vi "peaks_old.vi"(8 "error in (no error)":errorcluster, 9 "List Parameter Fit in":dbl[][](array[numeric]), 10 "List ROI in":dbl[][](array[numeric]), 11 "Spectrum In":cluster{"Locations":dbl[], "Amplitudes":dbl[]}[](array[cluster])=[{"Locations"=array[8192 elements], "Amplitudes"=array[8192 elements]}, {"Locations"=[0.7467606671708176, 1.9235641208245904, 2.29844815204634, 2.952058877083534, 3.30159027268929, 3.693510427204611, 4.0114062030881295, 5.465964569482503, 5.90533601872882, 6.405158056693529, 7.048430896937822, 7.965886489214608, 8.618241797175692, 9.551852093117594, 10.52313535167255, 11.040953037461485, 11.06991514504198, 11.223209663036432, 12.573413841890297, 13.028543500140618, 13.063940211907648, 13.079189646232502, 13.092703597511122, 13.151136366155567, 13.270484104491407, 13.336875706360313, 14.056987568841034, 14.657535881569391, 15.704563469510273, 16.589800479761752, 17.294355204547227, 18.547875406033366, 19.386017685106246, 23.796403305697343, 24.246601838900926, 24.938407230371723], "Amplitudes"=[8249.877716133802, 11327.172305519029, 56622.259938185096, 7573.210585087449, 5296.252862567521, 568942.2217447343, 85362.57126615923, 5991.635098339018, 7019.466820603001, 22054.8389595985, 7981.806397770608, 3443.0618845857953, 7232.474442522111, 1041.175508376075, 20253.913652049327, 2798.643385245958, 2822.1764574507447, 2760.065665975324, 27847.958569595598, 7072.034132274657, 7057.281156133169, 7080.033735934979, 7084.174530276932, 7080.4596184742295, 7256.269557996548, 7151.769553474873, 10957.376602343933, 8796.257531749367, 4885.946335626738, 151185.40382805822, 73397.38735258923, 16617.278737895518, 11305.024780412065, 1494.0162050533122, 1876.7337579234295, 12601.308465489856]}]) -> (0 "Error Out":errorcluster, 1 "List ROI out":dbl[][](array[numeric]), 2 "Table":string[][](table), 3 "Peaks Out":cluster{"Locations":dbl[], "Amplitudes":dbl[]}, 4 "List Parameter Fit Out":dbl[][](array[numeric]), 6 "Spectrum Fitted":cluster{"Array":dbl[], "Array":dbl[]})   [LabVIEW 2020]
uses:
  <vilib>/Utility/miscctls.llb/LVCursorListTypeDef.ctl
  b6f9e8ca-7105-a144-8367-28ac801578dd.vi
  85740291-8aab-ac43-b547-174ae308998b.vi
  01ce4f70-08cd-4644-9d74-9876cc86ca53.vi
  <vilib>/Utility/cursorutil.llb/Set Cursor (Icon Pict).vi
  control/global name path.vi
  <vilib>/Utility/Data Type/Get Array Information.vi
  <vilib>/Utility/Data Type/Get Type Information.vi
  <vilib>/Utility/file.llb/Write Delimited Spreadsheet (DBL).vi
  <vilib>/Utility/file.llb/Write Delimited Spreadsheet (string).vi
  <vilib>/Utility/file.llb/Read Delimited Spreadsheet (string).vi
  <vilib>/Utility/file.llb/Read Delimited Spreadsheet (DBL).vi
panel:
  in  "Fit":bool
  in  "mapping":u16(ring) items=["Y - Linear", "Y - Log"]
  out "CrsrList":T1(array[cluster])
  in  "Open":bool
  in  "Save":bool
  in  "eval":bool
  in  "custom":bool
  out "cluster roi":T2
  out "element":cluster{"Locations":dbl[], "Amplitudes":dbl[]}
  out "Cursor Name":string
  in  "Reset":bool
  out "Array":dbl[][](array[numeric])
  out "removing":bool
  in  "Normal":bool
  in  "Remove":bool
  in  "Cursor Icon":u16(ring)
  in  "Stop Button":bool
  out "Spectrum":cluster{"Locations":dbl[], "Amplitudes":dbl[]}[](graph)=[{"Locations"=array[8192 elements], "Amplitudes"=array[8192 elements]}, {"Locations"=[0.6846487923218129, 0.8031614293624534, 1.7242543828557408, 1.938747247460668, 2.306953300257028, 2.6210970168759666, 2.9711981229526625, 3.3277824164248653, 3.7170873790620336, 4.04405224728037, 6.436481431667202, 7.096967343713246, 7.460990586502177, 7.523333804369678, 7.617042760860395, 8.127017296174136, 8.194901838112248, 8.297705547082785, 8.30569855209705, 8.683571266368165, 9.291525652441827, 9.336316527839342, 9.702473642891427, 10.164949159251092, 10.940151266361038, 10.984300604976537, 11.073242471735028, 11.160271165263742, 11.268603021790387, 11.368683422279902, 11.476870860603926, 11.732338216351955, 11.74047488132859, 11.913527841198139, 12.313442472513525, 12.422414883693174, 12.679357859240612, 13.137181465596367, 13.560377222755834, 13.985871403462042, 14.181757913002619, 14.811990689785183, 15.123878999537014, 15.225144239474576, 15.847402751701654, 15.936506376474796, 15.997115442383588, 16.751668923733696, 17.456338945421972, 18.685517095107702, 19.565242039112338, 23.10994450808025, 23.25953036719509, 23.37377015691927, 23.439242722748002, 23.98629158276466, 24.428149293414577, 24.684829964850557, 24.772035910147434, 25.173301655535283], "Amplitudes"=[5749.475271060954, 5002.0142432044795, 4437.978004734703, 11660.526656612647, 65746.84001208292, 2894.387213953257, 9849.360532927198, 7160.035072829482, 645601.7858592308, 95492.33538323875, 14805.060779816191, 1620.7095092057602, 1146.3915335122922, 1168.4930336372568, 1322.5033864359928, 4245.563045439152, 4184.35157964611, 4422.765014063421, 4401.872906279167, 13740.871473164421, 12716.350040257696, 12964.336303896753, 16789.033949154484, 20702.823823277406, 27073.790223214626, 26827.13611017004, 26877.36292640188, 26681.744011808405, 26623.286988764616, 26394.35650952068, 26015.737537837078, 23980.0092551179, 23996.924012643343, 23101.773776484937, 20651.803398511016, 20229.386024779047, 41284.21044656313, 13637.881570622103, 8980.093476318705, 5646.466867551864, 7355.058688359613, 4885.822952660352, 292.0377308174795, 694.6108290767994, 6797.9436035222725, 6852.18604910736, 6738.9197496309225, 156943.61193784876, 77075.8593535495, 10701.96206664513, 3415.986171238152, 30.039025289396076, 37.780232933378514, 78.71549190995782, 52.215114100379424, 895.4437472888932, 1309.544166875224, 1288.517058471017, 1383.105839373177, 18123.868845544213]}]
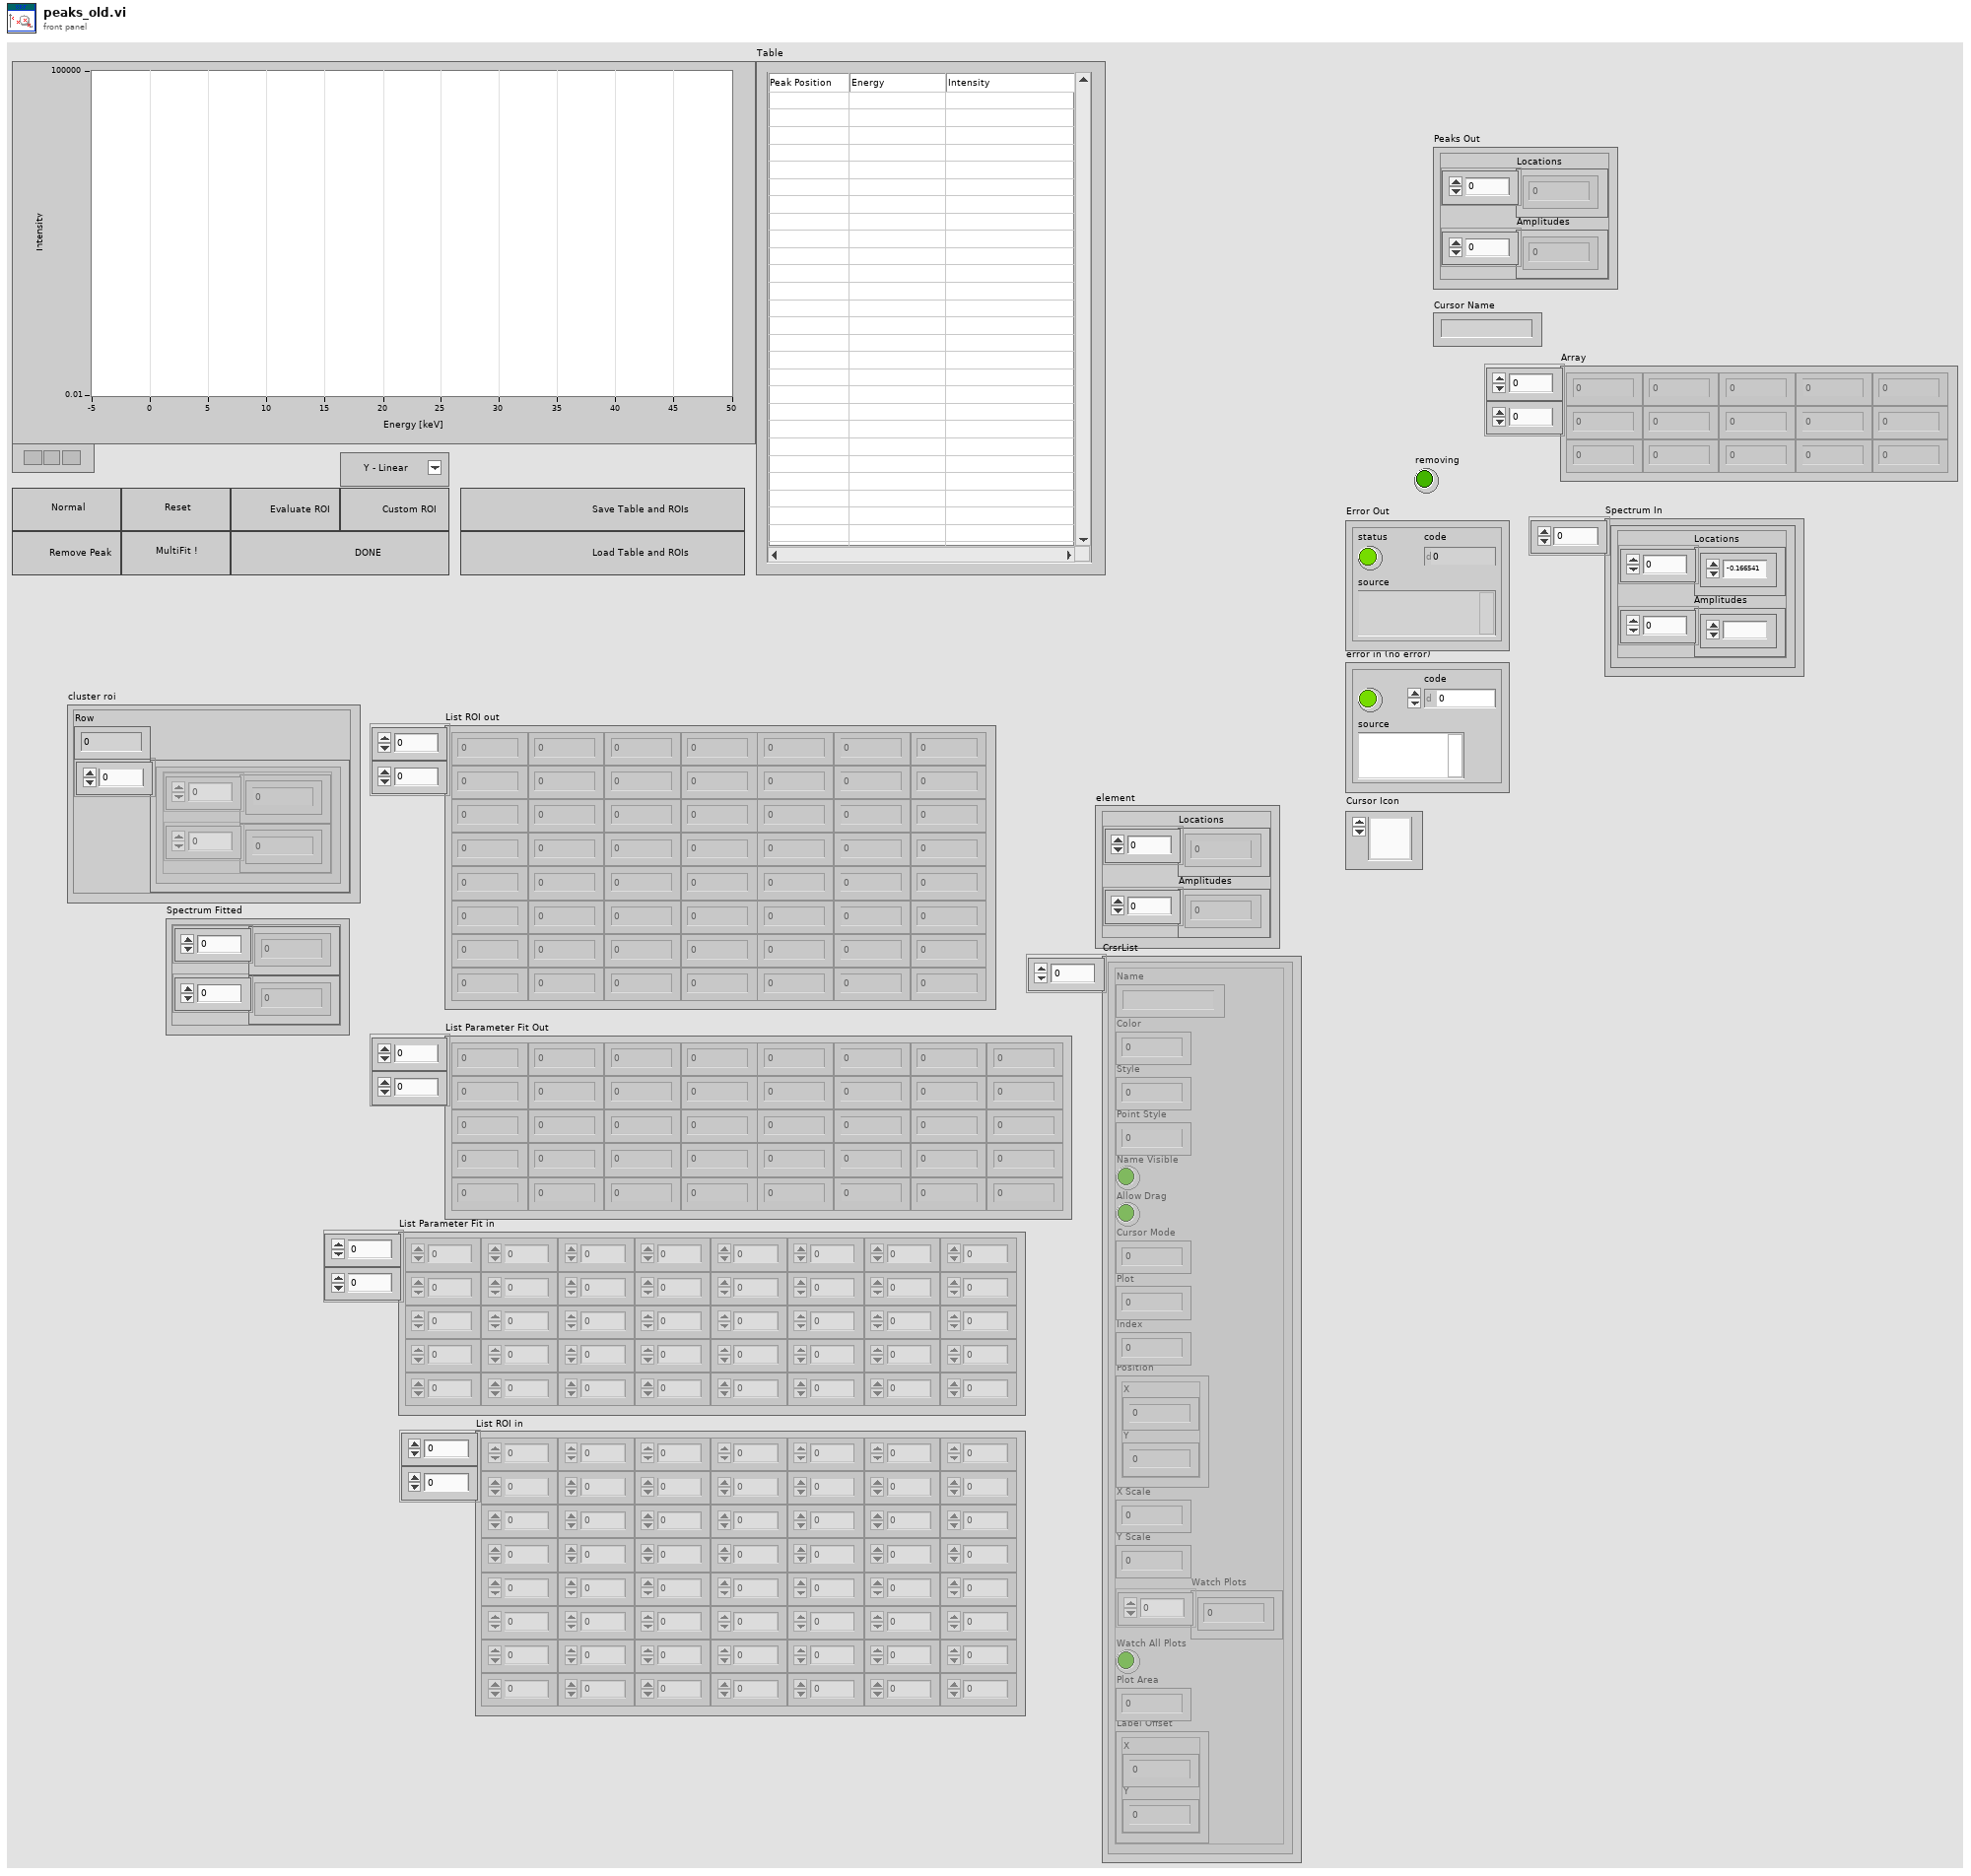
[diagram p1: front panel]
types:
  T1 = cluster{"Name":string, "Color":u32, "Style":i32, "Point Style":i32, "Name Visible":bool, "Allow Drag":bool, "Cursor Mode":u32, "Plot":i32, "Index":i32, "Position":cluster{"X":dbl, "Y":dbl}, "X Scale":u32, "Y Scale":u32, "Watch Plots":i32[], "Watch All Plots":bool, "Plot Area":i32, "Label Offset":cluster{"X":dbl, "Y":dbl}}[]
  T2 = cluster{"Row":i32, "Array":cluster{"Array":dbl[], "Array":dbl[]}[]}
  T3 = typedef "LVCursorListTypeDef.ctl" = cluster{"Name":string, "Color":u32, "Style":u8, "Point Style":u8, "Name Visible":bool, "Allow Drag":bool, "Cursor Mode":u32, "Plot":i32, "Index":i32, "Position":cluster{"X":dbl, "Y":dbl}, "X Scale":u32, "Y Scale":u32, "Watch Plots":i32[], "Watch All Plots":bool, "Plot Area":i32, "Label Offset":cluster{"X":dbl, "Y":dbl}}[]
  T4 = cluster{"Name":string, "Color":u32, "Style":i32, "Point Style":i32, "Name Visible":bool, "Allow Drag":bool, "Cursor Mode":u32, "Plot":i32, "Index":i32, "Position":cluster{"X":dbl, "Y":dbl}, "X Scale":u32, "Y Scale":u32, "Watch Plots":i32[], "Watch All Plots":bool, "Plot Area":i32, "Label Offset":cluster{"X":dbl, "Y":dbl}}
  T5 = typedef "LVPoint32TypeDef.ctl" = cluster{"Horizontal":i32, "Vertical":i32}
  T6 = typedef "LVRowAndColumnTypeDef.ctl" = cluster{"Row":i32, "Column":i32}
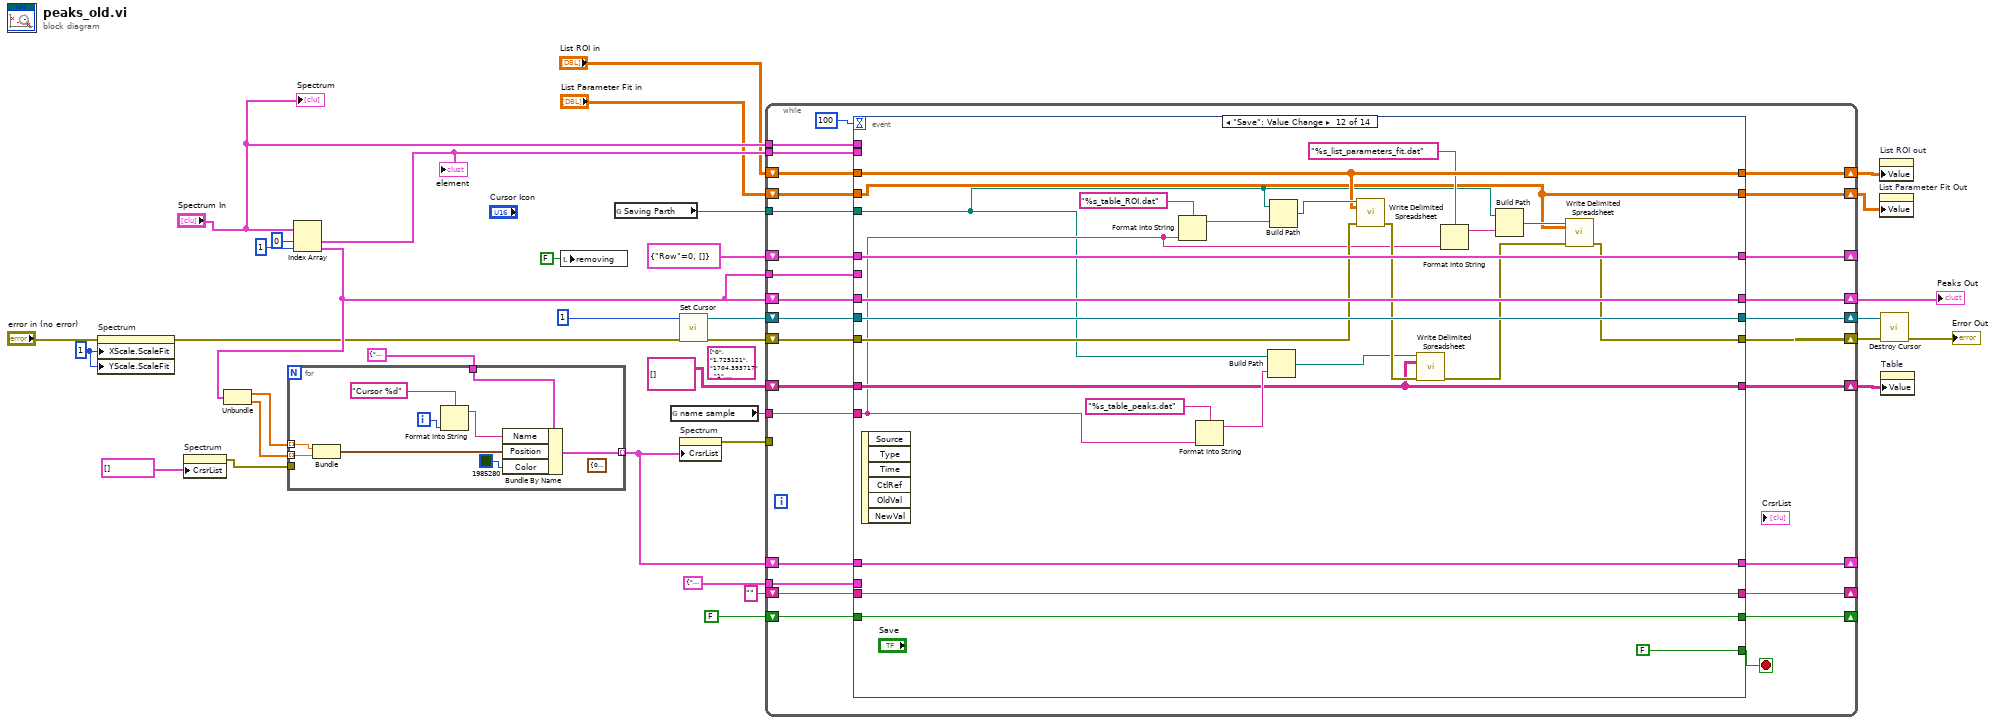
[diagram p0: block diagram]
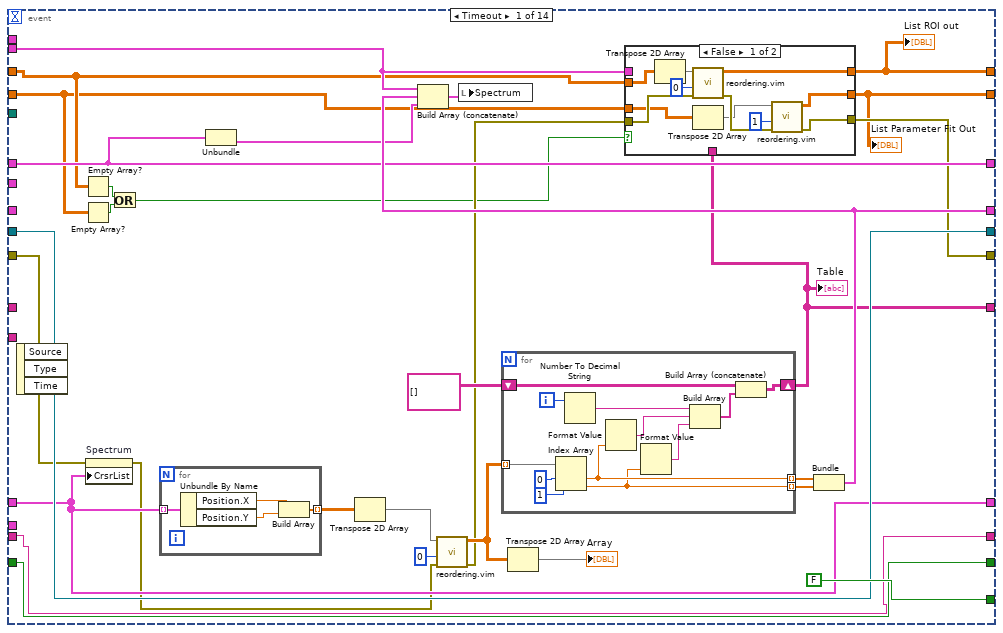
[diagram p2: hidden frame]
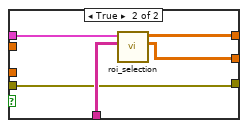
[diagram p3: hidden frame]
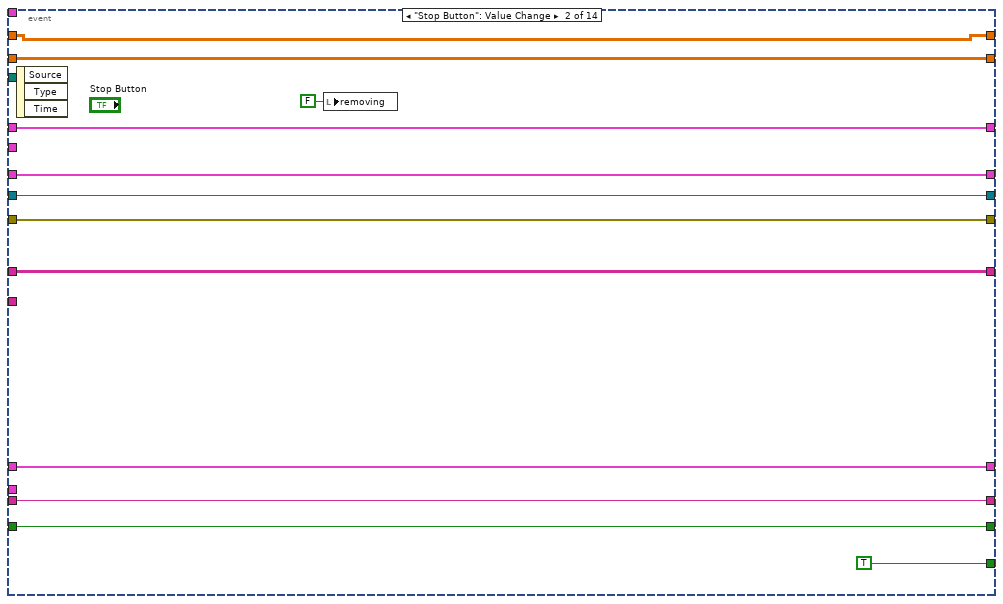
[diagram p4: hidden frame]
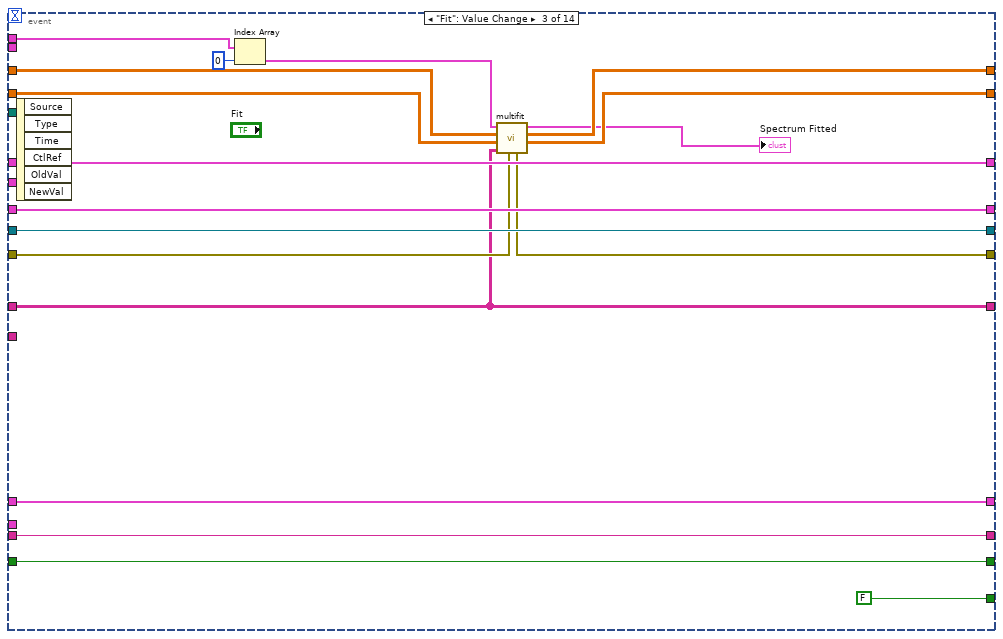
[diagram p5: hidden frame]
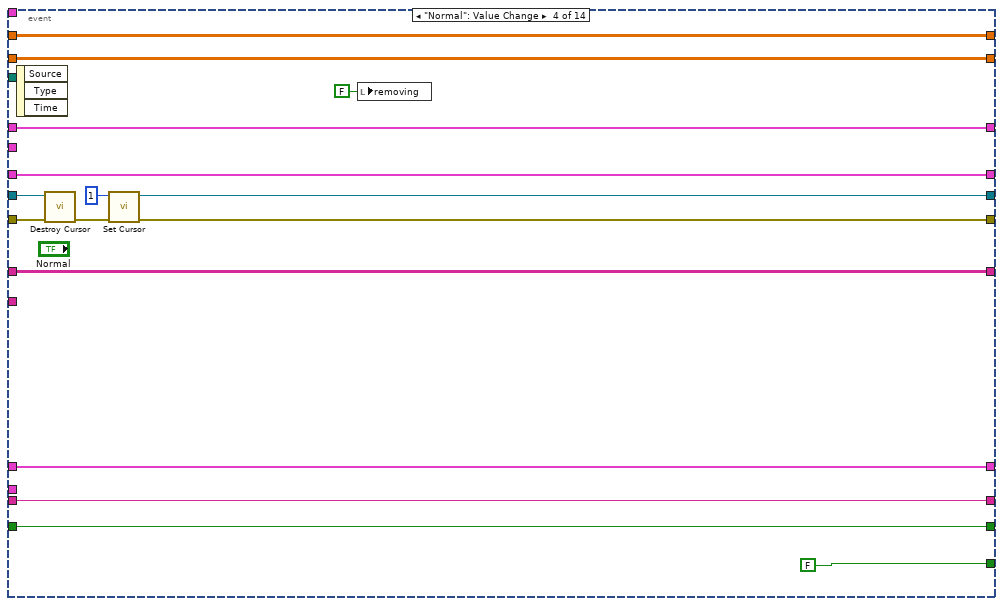
[diagram p6: hidden frame]
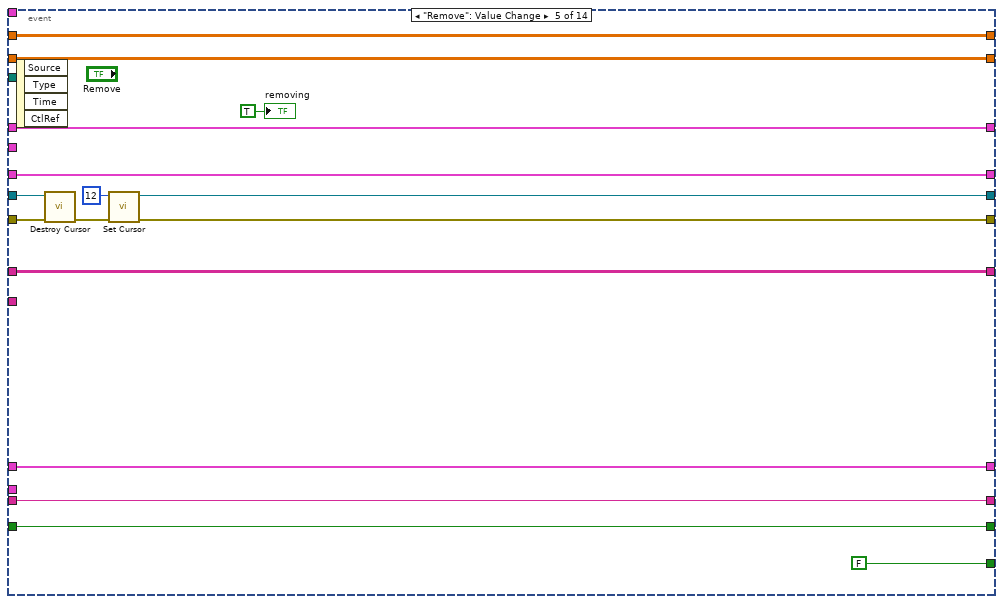
[diagram p7: hidden frame]
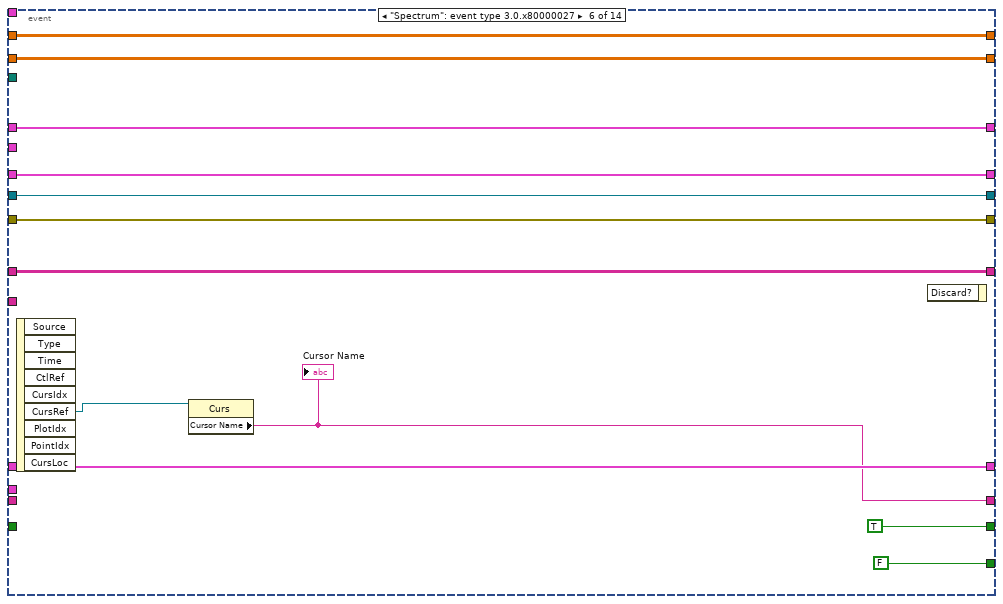
[diagram p8: hidden frame]
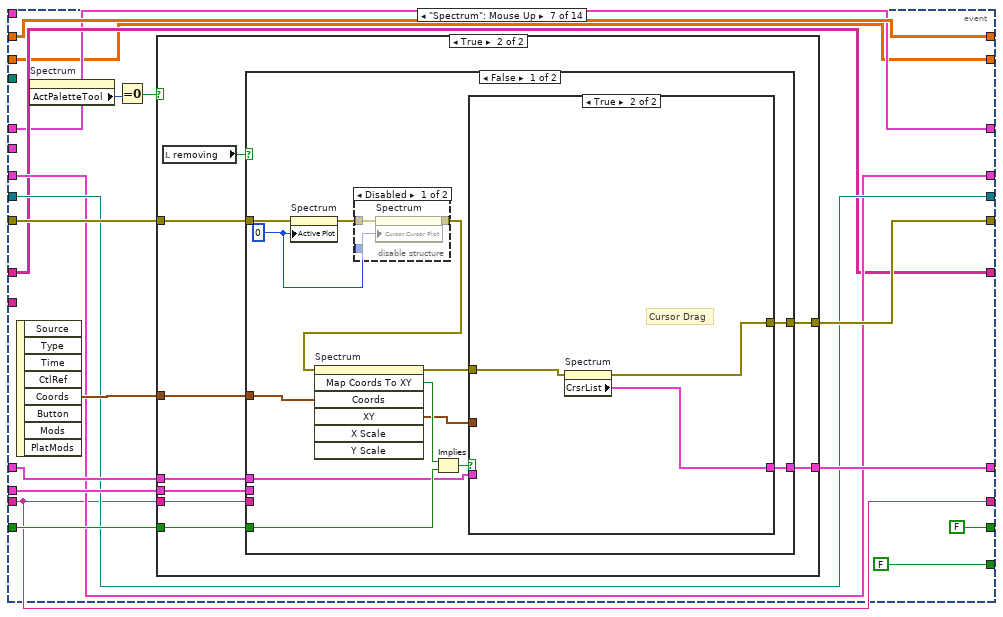
[diagram p9: hidden frame]
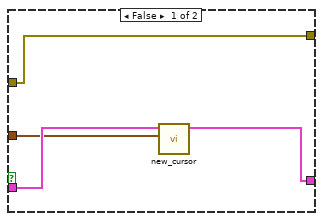
[diagram p12: hidden frame]
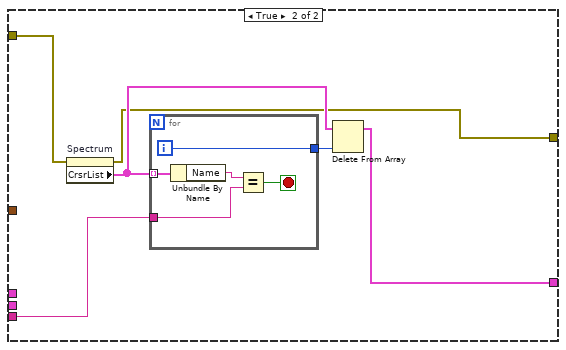
[diagram p13: hidden frame]
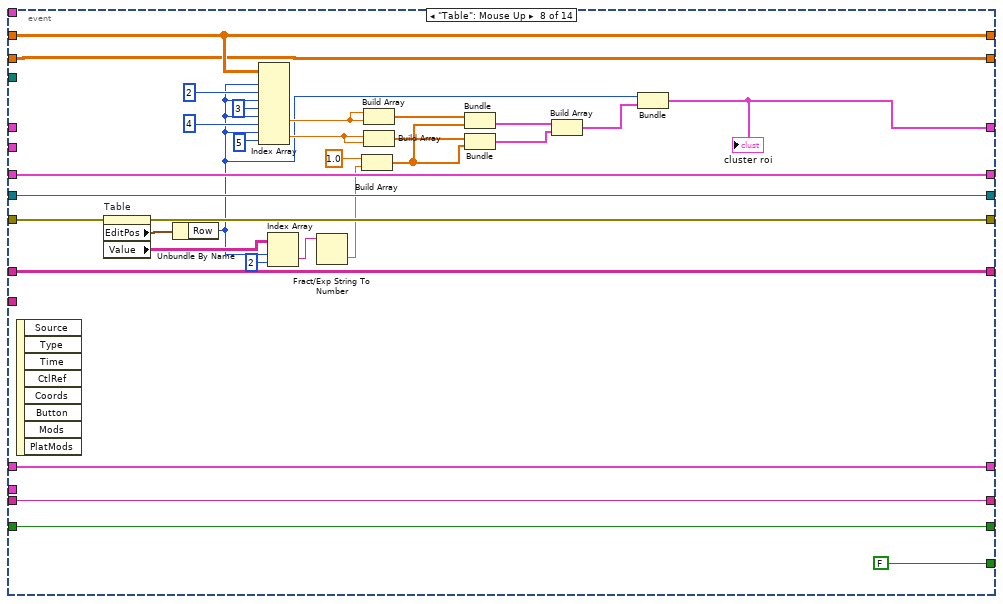
[diagram p14: hidden frame]
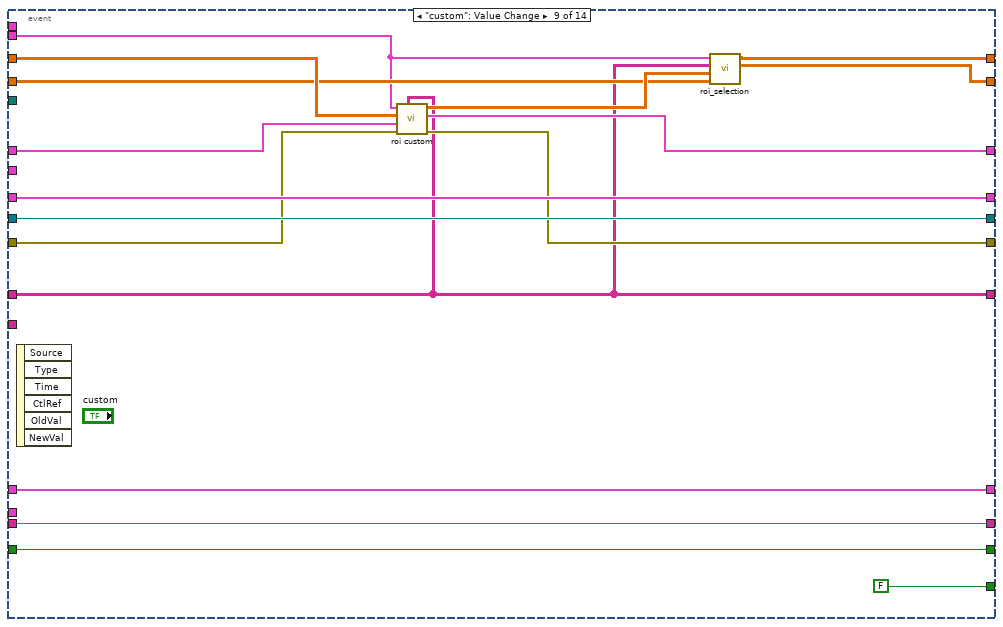
[diagram p15: hidden frame]
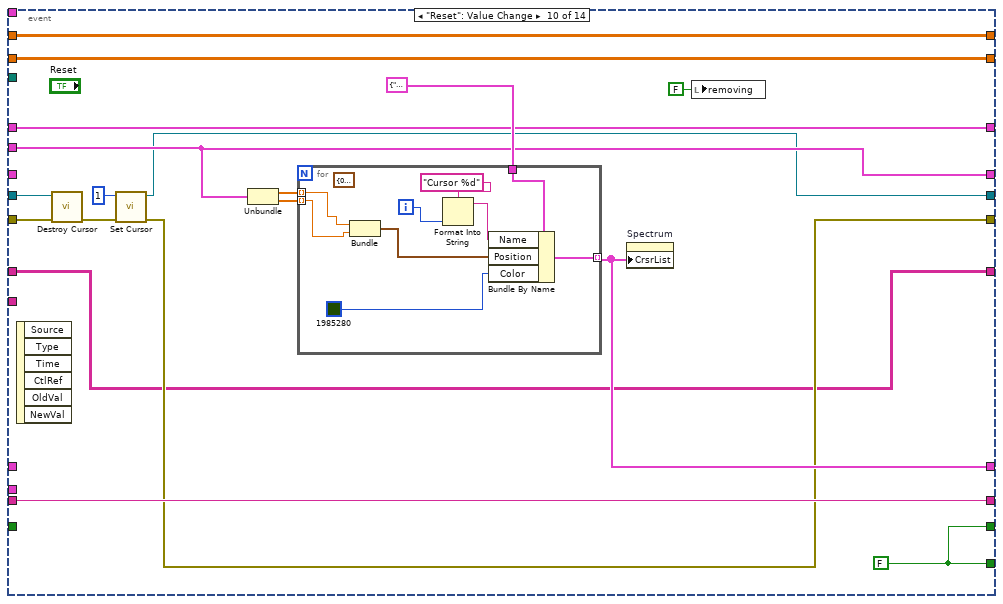
[diagram p16: hidden frame]
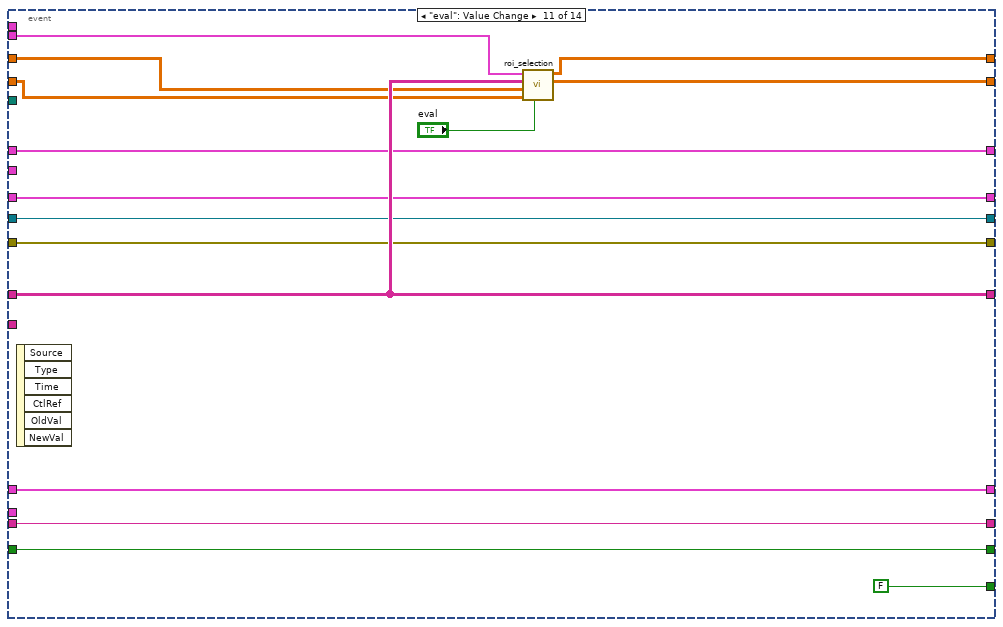
[diagram p17: hidden frame]
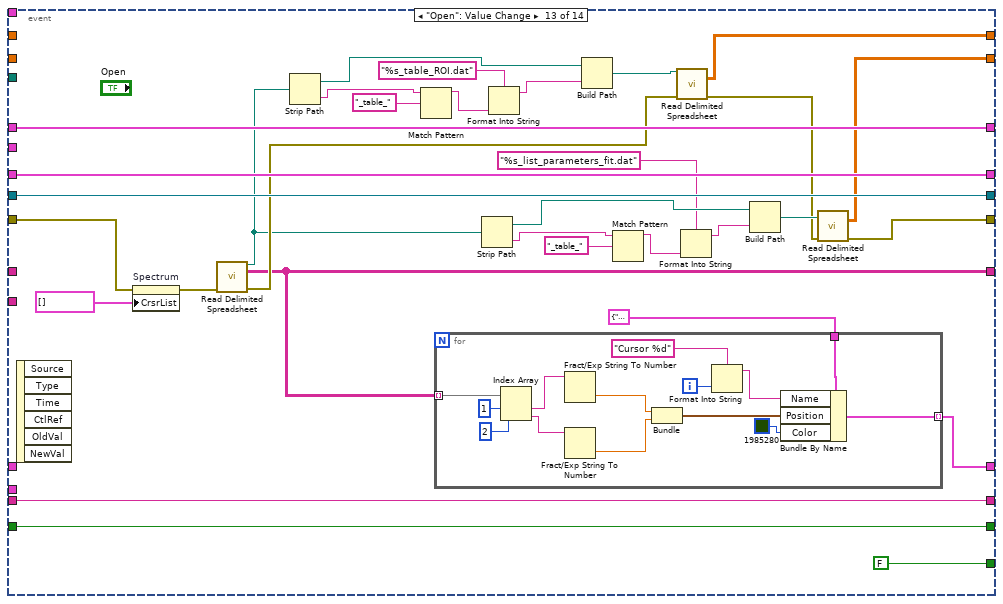
[diagram p18: hidden frame]
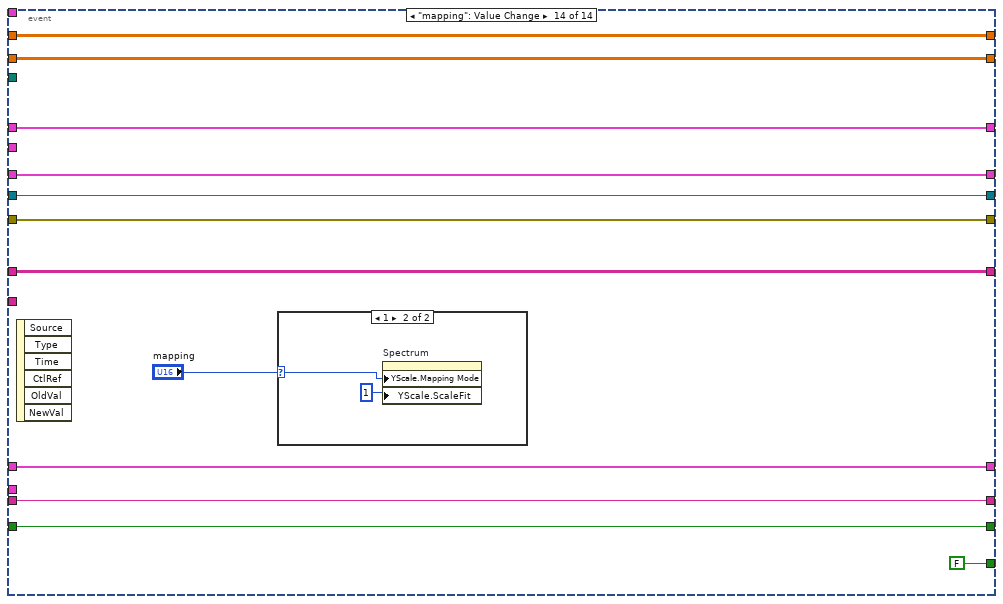
[diagram p19: hidden frame]
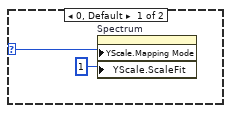
[diagram p20: hidden frame]
diagram:
  w11 = u8 1 ("X Scale.Scale Fit")
  (unwired) string[][] [["0", "1.725121", "1704.393717"], ["1", "1.970845", "984.228481"], ["2", "2.303441", "1944.031171"], ["3", "2.614035", "2011.669918"], ["4", "2.952544", "4620.007915"], ["5", "3.307548", "9783.329806"], ["6", "3.691265", "30769.779466"], ["7", "4.014453", "4616.583275"], ["8", "4.510204", "698.422233"], ["9", "4.927114", "412.615986"], ["10", "5.950437", "698.422233"], ["11", "6.402564", "4117.128631"], ["12", "8.072886", "984.228481"], ["13", "8.615424", "2806.402012"], ["14", "10.509461", "8738.084886"], ["15", "12.556457", "12119.486590"], ["16", "14.027261", "5340.202284"], ["17", "14.636488", "4362.343076"]] ("Table")
  n1 = property on="Spectrum" class="XYGraph (strict)"(error in="error in (no error)", "XScale.ScaleFit"=w11, "YScale.ScaleFit"=w11) -> (error out=w9:errorcluster)  [unwired: 1 in, 1 out]
  n2 = property on="Spectrum" class="XYGraph (strict)"("CrsrList"=T3 [] ("Cursor List")) -> (error out=w21:errorcluster)  [unwired: 2 in, 1 out]
  n3 = Index Array(array="Spectrum In", index #1=0 ("index"), index #2=1 ("index")) -> (element #1=w15:cluster{"Locations":dbl[], "Amplitudes":dbl[]}, element #2=w17:cluster{"Locations":dbl[], "Amplitudes":dbl[]})
  "element" <- w15
  n4 = Unbundle(w17) -> ("Locations"=w25:dbl[], "Amplitudes"=w24:dbl[])
  n5 = for {
    tunnel: w25 -> [w42] mode=indexing
    tunnel: w24 -> [w41] mode=indexing
    tunnel: T4 {"Name"="", "Color"=16776704, "Style"=4, "Point Style"=13, "Name Visible"=FALSE, "Allow Drag"=TRUE, "Cursor Mode"=0, "Plot"=0, "Index"=0, "Position"={"X"=0.0, "Y"=0.0}, "X Scale"=0, "Y Scale"=0, "Watch Plots"=[], "Watch All Plots"=FALSE, "Plot Area"=0, "Label Offset"={"X"=0.0, "Y"=0.0}} -> [w40]
    tunnel: w21 -> [_]
    tunnel: [w36] -> w18 mode=indexing
    i -> [w43]
    (unwired) cluster{"X":dbl, "Y":dbl} {"X"=0.0, "Y"=0.0} ("XY")
    n6 = Bundle("Numeric Control"=w42, "Numeric"=w41) -> (w37:cluster{"Numeric Control":dbl, "Numeric":dbl})  [unwired: 1 in]
    n7 = Format Into String(format string="Cursor %d", w43) -> (resulting string=w39:string)  [unwired: 2 in, 1 out]
    n8 = Bundle By Name(cluster=w40, "Name"=w39, "Position"=w37, "Color"=u32 1985280) -> (w36:T4)
  }
  n9 = local write "removing"(FALSE ("removing")) -> ()
  n10 = global read "global name path.vi" "Saving Parth"() -> (w2:path)
  n11 = global read "global name path.vi" "name sample"() -> (w1:string)
  n12 = call-poly <vilib>:"Set Cursor.vi"("error in (no error)"=w9, "icon"=u16 1 ("Cursor Icon")) -> ("error out"=w32:errorcluster, "previous cursor ID"=w33:refnum<k1>)  [unwired: 8 in]
  n13 = property on="Spectrum" class="XYGraph (strict)"("CrsrList"=w18) -> (error out=w20:errorcluster)  [unwired: 2 in, 1 out]
  n14 = while {
    shift-right: [w71] -> w31
    shift-left: w32 -> [w70]
    shift-right: [w68] -> w29
    shift-left: w33 -> [w69]
    shift-right: [w66] -> w16
    shift-left: w17 -> [w67]
    shift-right: [w65] -> _
    shift-left: FALSE -> [w64]
    tunnel: T4 {"Name"="", "Color"=16776704, "Style"=4, "Point Style"=13, "Name Visible"=FALSE, "Allow Drag"=TRUE, "Cursor Mode"=0, "Plot"=0, "Index"=0, "Position"={"X"=0.0, "Y"=0.0}, "X Scale"=0, "Y Scale"=0, "Watch Plots"=[], "Watch All Plots"=FALSE, "Plot Area"=0, "Label Offset"={"X"=0.0, "Y"=0.0}} -> [w63]
    shift-right: [w61] -> _
    shift-left: w18 -> [w62]
    tunnel: w20 -> [_]
    shift-right: [w59] -> _
    shift-left: "" ("Cursor Name") -> [w58]
    tunnel: w17 -> [w57]
    shift-right: [w55] -> w5
    shift-left: string[][] [] ("Table") -> [w54]
    shift-right: [w53] -> w7
    shift-left: "List ROI in" -> [w52]
    tunnel: w15 -> [w56]
    shift-right: [w51] -> _
    shift-left: cluster{"Row":i32, cluster{dbl[], dbl[]}[]} {"Row"=0, []} -> [w50]
    shift-right: [w49] -> w6
    shift-left: "List Parameter Fit in" -> [w48]
    tunnel: "Spectrum In" -> [w47]
    tunnel: w2 -> [w46]
    tunnel: w1 -> [w45]
    stop <- w72 stop-if-true
    n15 = event shown="[11] \"Save\": Value Change" {
      selector: _ -> [_ _ _ _ _ _ _ _ _ _ _ _ _ _]
      dyn-events: _ -> [_ _ _ _ _ _ _ _ _ _ _ _ _ _]
      timeout: 100 -> [_ _ _ _ _ _ _ _ _ _ _ _ _ _]
      tunnel: [FALSE TRUE FALSE FALSE FALSE FALSE FALSE FALSE FALSE w321 FALSE FALSE FALSE FALSE] -> w72
      tunnel: [w82 w138 w156 w176 w192 w207 w220 w296 w312 w327 w355 w364 w388 w439] -> w71
      tunnel: w70 -> [w80 w138 w157 w180 w196 w207 w219 w297 w311 w328 w355 w374 w398 w439]
      tunnel: w69 -> [w101 w145 w163 w179 w195 w206 w218 w299 w315 w325 w356 w383 w415 w438]
      tunnel: [w101 w145 w163 w175 w191 w206 w218 w299 w315 w326 w356 w383 w415 w438] -> w68
      tunnel: w67 -> [_ w144 w162 w173 w189 w205 w217 w298 w314 _ w357 w382 w414 w437]
      tunnel: [w91 w144 w162 w173 w189 w205 w217 w298 w314 w334 w357 w382 w414 w437] -> w66
      tunnel: [w100 w143 w161 w172 w188 TRUE FALSE w300 w317 w321 w352 w385 w416 w442] -> w65
      tunnel: w64 -> [w100 w143 w161 w172 w188 _ w224 w300 w317 _ w352 w385 w416 w442]
      tunnel: w63 -> [_ _ _ _ _ _ w223 _ _ _ _ _ _ _]
      tunnel: w62 -> [w81 w142 w160 w171 w187 w203 w222 w288 w319 _ w354 w384 _ w444]
      tunnel: [w81 w142 w160 w171 w187 w203 w221 w288 w319 w332 w354 w384 w401 w444] -> w61
      tunnel: [w89 w139 w158 w166 w182 w201 w211 w301 w316 w331 w353 w370 w417 w443] -> w59
      tunnel: w58 -> [w89 w139 w158 w166 w182 _ w211 w301 w316 w331 w353 w370 w417 w443]
      tunnel: w57 -> [_ _ _ _ _ _ _ _ _ w334 _ _ _ _]
      tunnel: w56 -> [w85 _ _ _ _ _ _ _ w303 _ w361 _ _ _]
      tunnel: [w84 w137 w148 w169 w185 w200 w214 w294 w304 w324 w360 w371 w403 w440] -> w55
      tunnel: w54 -> [_ w137 w148 w169 w185 w200 w214 w294 w304 w324 w360 w371 _ w440]
      tunnel: [w86 w136 w152 w168 w184 w199 w213 w293 w305 w323 w359 w375 w405 w435] -> w53
      tunnel: w52 -> [w75 w136 w155 w168 w184 w199 w213 w293 w313 w323 w349 w375 _ w435]
      tunnel: [w88 w140 w159 w167 w183 w198 w212 w273 w309 w322 w358 w381 w413 w436] -> w51
      tunnel: w50 -> [w88 w140 w159 w167 w183 w198 w212 _ w310 w322 w358 w381 w413 w436]
      tunnel: w45 -> [_ _ _ _ _ _ _ _ _ _ _ w368 _ _]
      tunnel: [w78 w135 w153 w165 w181 w197 w209 w272 w306 w320 w350 w363 w387 w433] -> w49
      tunnel: w48 -> [w74 w135 w154 w165 w181 w197 w209 w272 w307 w320 w348 w363 _ w433]
      tunnel: w47 -> [_ _ w151 _ _ _ _ _ _ _ _ _ _ _]
      tunnel: w46 -> [_ _ _ _ _ _ _ _ _ _ _ w362 _ _]
      event Timeout {
        n16 = event-data() -> ()  [unwired: 1 in, 3 out]
        n17 = Empty Array?(array=w75) -> (empty?=w77:bool)
        n18 = Empty Array?(array=w74) -> (empty?=w76:bool)
        n19 = property on="Spectrum" class="XYGraph (strict)"(error in=w80, "CrsrList"=w81) -> (error out=w79:errorcluster)  [unwired: 1 in, 1 out]
        n20 = Or(x=w77, y=w76) -> (x .or. y?=w73:bool)
        n21 = for {
          tunnel: w81 -> [w134] mode=indexing
          tunnel: [w131] -> w99 mode=indexing
          n22 = Unbundle By Name(w134) -> ("Position.X"=w133:dbl, "Position.Y"=w132:dbl)
          n23 = Build Array(w133, w132) -> (w131:dbl[])
        }
        n24 = Unbundle(w88) -> (w87:cluster{dbl[], dbl[]}[])  [unwired: 1 out]
        n25 = Transpose 2D Array(2D array=w99) -> (transposed array=w98:dbl[][])
        n26 = call "reordering.vim"("error in (no error)"=w79, "Row to Reorder"=0, "Data In"=w98) -> ("Error Out"=w83:errorcluster, "Data Out"=w95:dbl[][])  [unwired: 7 in]
        n27 = for {
          tunnel: w95 -> [w130] mode=indexing
          tunnel: [w126] -> w94 mode=indexing
          tunnel: [w125] -> w93 mode=indexing
          shift-right: [w119] -> w84
          shift-left: string[][] [] ("Table") -> [w121]
          i -> [w127]
          n28 = Index Array(array=w130, index #1=0 ("index"), index #2=1 ("index")) -> (element #1=w126:dbl, element #2=w125:dbl)
          n29 = Number To Decimal String(number=w127) -> (decimal integer string=w122:string)  [unwired: 1 in]
          n30 = Format Value(value (0)=w126) -> (output string=w123:string)  [unwired: 2 in]
          n31 = Format Value(value (0)=w125) -> (output string=w124:string)  [unwired: 2 in]
          n32 = Build Array(w122, w123, w124) -> (w120:string[])
          n33 = Build Array (concatenate)(w121, w120) -> (w119:string[][])
        }
        "Table" <- w84
        n34 = Transpose 2D Array(2D array=w95) -> (transposed array=→"Array":dbl[][])
        n35 = case shown="False" w73 {
          tunnel: [w110 w118] -> w86
          tunnel: w85 -> [_ w117]
          tunnel: w84 -> [_ w116]
          tunnel: w75 -> [w111 _]
          tunnel: w83 -> [w109 w115]
          tunnel: [w104 w115] -> w82
          tunnel: w74 -> [w108 _]
          tunnel: [w103 w114] -> w78
          frame False {
            n36 = Transpose 2D Array(2D array=w111) -> (transposed array=w113:dbl[][])
            n37 = call "reordering.vim"("error in (no error)"=w109, "Row to Reorder"=0, "Data In"=w113) -> ("Error Out"=w107:errorcluster, "Data Out"=w110:dbl[][])  [unwired: 7 in]
            n38 = Transpose 2D Array(2D array=w108) -> (transposed array=w106:dbl[][])
            n39 = call "reordering.vim"("error in (no error)"=w107, "Row to Reorder"=1, "Data In"=w106) -> ("Error Out"=w104:errorcluster, "Data Out"=w103:dbl[][])  [unwired: 7 in]
          }
          frame True {
            n40 = call "roi_selection.vi"("List Peaks"=w116, "Spectrum In"=w117) -> ("List Parameter Fit Out"=w114:dbl[][], "List ROI Out"=w118:dbl[][])  [unwired: 8 in]
          }
        }
        "List ROI out" <- w86
        "List Parameter Fit Out" <- w78
        n41 = Bundle(w94, w93) -> (w91:cluster{dbl[], dbl[]})  [unwired: 1 in]
        n42 = Build Array (concatenate)(w85, w91, w87) -> (w90:cluster{"Locations":dbl[], "Amplitudes":dbl[]}[])
        n43 = local write "Spectrum"(w90) -> ()
      }
      event "Stop Button": Value Change {
        n44 = event-data() -> ()  [unwired: 1 in, 3 out]
        n45 = local write "removing"(FALSE ("removing")) -> ()
      }
      event "Fit": Value Change {
        n46 = event-data() -> ()  [unwired: 1 in, 6 out]
        n47 = Index Array(array=w151, index=0) -> (element=w149:cluster{"Locations":dbl[], "Amplitudes":dbl[]})
        n48 = call "multifit.vi"("error in"=w157, "List Peaks"=w148, "List Parameter Fit In"=w154, "List ROI In"=w155, "Spectrum In"=w149) -> ("List Parameter Fit Out"=w153:dbl[][], "List ROI Out"=w152:dbl[][], "Spectrum Fitted"=→"Spectrum Fitted":cluster{"Array":dbl[], "Array":dbl[]}, "error out"=w156:errorcluster)  [unwired: 3 in]
      }
      event "Normal": Value Change {
        n49 = event-data() -> ()  [unwired: 1 in, 3 out]
        n50 = call <vilib>:"Destroy Cursor.vi"("cursor ID"=w179, "error in (no error)"=w180) -> ("error out"=w178:errorcluster)  [unwired: 8 in]
        n51 = call-poly <vilib>:"Set Cursor.vi"("error in (no error)"=w178, "icon"=u16 1 ("Cursor Icon")) -> ("error out"=w176:errorcluster, "previous cursor ID"=w175:refnum<k1>)  [unwired: 8 in]
        n52 = local write "removing"(FALSE ("removing")) -> ()
      }
      event "Remove": Value Change {
        n53 = event-data() -> ()  [unwired: 1 in, 4 out]
        n54 = call <vilib>:"Destroy Cursor.vi"("cursor ID"=w195, "error in (no error)"=w196) -> ("error out"=w194:errorcluster)  [unwired: 8 in]
        n55 = call-poly <vilib>:"Set Cursor.vi"("error in (no error)"=w194, "icon"=u16 12 ("Cursor Icon")) -> ("error out"=w192:errorcluster, "previous cursor ID"=w191:refnum<k1>)  [unwired: 8 in]
        "removing" <- TRUE ("removing")
      }
      event "Spectrum": event type 3.0.x80000027 {
        n56 = event-data() -> ("CursRef"=w202:refnum<vi>)  [unwired: 1 in, 8 out]
        n57 = property class="Curs"(reference=w202) -> ("Cursor Name"=w201:string)  [unwired: 1 in, 2 out]
        "Cursor Name" <- w201
        n58 = event-data() -> ()  [unwired: 2 in, 1 out]
      }
      event "Spectrum": Mouse Up {
        n59 = event-data() -> ("Coords"=w225:T5)  [unwired: 1 in, 7 out]
        n60 = property on="Spectrum" class="XYGraph (strict)"() -> ("ActPaletteTool"=w216:i32)  [unwired: 2 in, 2 out]
        n61 = Equal To 0?(x=w216) -> (x = 0?=w215:bool)
        n62 = case shown="True" w215 {
          tunnel: w225 -> [_ w237]
          tunnel: w224 -> [_ w236]
          tunnel: w223 -> [_ w235]
          tunnel: w222 -> [w227 w234]
          tunnel: [w227 w232] -> w221
          tunnel: [w228 w231] -> w220
          tunnel: w219 -> [w228 w230]
          tunnel: w211 -> [_ w229]
          frame False {
          }
          frame True {
            n63 = local read "removing"() -> (w233:bool)
            n64 = case shown="False" w233 {
              tunnel: w237 -> [w250 _]
              tunnel: w236 -> [w248 _]
              tunnel: w235 -> [_ _]
              tunnel: w234 -> [w245 _]
              tunnel: [w244 w263] -> w232
              tunnel: w229 -> [_ w266]
              tunnel: [w242 w261] -> w231
              tunnel: w230 -> [w241 w262]
              frame False {
                w238 = u32 0 ("Active Plot")
                n65 = property on="Spectrum" class="XYGraph (strict)"(error in=w241, "Active Plot"=w238) -> (error out=w240:errorcluster)  [unwired: 1 in, 1 out]
                n66 = disable-structure shown="Disabled" {
                  disable-tunnel: w240 -> [w253 _]
                  disable-tunnel: [w252 _] -> w239
                  disable-tunnel: w238 -> [w251 _]
                  frame Disabled {
                    n67 = property on="Spectrum" class="XYGraph (strict)"(error in=w253, "Cursor.Cursor Plot"=w251) -> (error out=w252:errorcluster)  [unwired: 1 in, 1 out]
                  }
                  frame Enabled {
                  }
                }
                n68 = invoke on="Spectrum" class="XYGraph (strict)" method="Map Coords To XY"(error in=w239, "Coords"=w250) -> (error out=w243:errorcluster, "Map Coords To XY"=w249:bool, "XY"=w246:cluster{"X":dbl, "Y":dbl})  [unwired: 5 in, 4 out]
                n69 = Implies(1:w248, 2:w249) -> (0:w247:bool)
                n70 = case shown="True" w247 {
                  tunnel: [w254 w260] -> w244
                  tunnel: w246 -> [w255 _]
                  tunnel: w245 -> [w256 _]
                  tunnel: w243 -> [w257 w259]
                  tunnel: [w257 w258] -> w242
                  frame False {
                    n71 = call "new_cursor.vi"("XY"=w255, "CrsrList"=w256) -> ("CrsrList Out"=w254:T1)  [unwired: 9 in]
                  }
                  frame True {
                    # "Cursor Drag"
                    n72 = property on="Spectrum" class="XYGraph (strict)"(error in=w259) -> (error out=w258:errorcluster, "CrsrList"=w260:T3)  [unwired: 1 in, 1 out]
                  }
                }
              }
              frame True {
                n73 = property on="Spectrum" class="XYGraph (strict)"(error in=w262) -> (error out=w261:errorcluster, "CrsrList"=w265:T3)  [unwired: 1 in, 1 out]
                n74 = for {
                  tunnel: w265 -> [w271] mode=indexing
                  tunnel: w266 -> [w269]
                  tunnel: [w267] -> w264
                  i -> [w267]
                  stop <- w268 stop-if-true
                  n75 = Unbundle By Name(w271) -> ("Name"=w270:string)
                  n76 = Equal?(x=w270, y=w269) -> (x = y?=w268:bool)
                }
                n77 = Delete From Array(array=w265, index=w264) -> (array with subset deleted=w263:T3)  [unwired: 1 in, 1 out]
              }
            }
          }
        }
      }
      event "Table": Mouse Up {
        n78 = event-data() -> ()  [unwired: 1 in, 8 out]
        n79 = property on="Table" class="Tbl (strict)"(error in=w297) -> (error out=w296:errorcluster, "EditPos"=w295:T6, "Value"=w287:string[][])  [unwired: 1 in, 1 out]
        n80 = Unbundle By Name(w295) -> ("Row"=w275:i32)
        n81 = Index Array(array=w293, index (row) #1=w275, index (col) #1=2 ("disabled index (col)"), index (row) #2=w275, index (col) #2=3 ("disabled index (col)"), index (row) #3=w275, index (col) #3=4 ("disabled index (col)"), index (row) #4=w275, index (col) #4=5 ("disabled index (col)")) -> (element #3=w283:dbl, element #4=w280:dbl)  [unwired: 2 out]
        n82 = Index Array(array=w287, index (row)=w275, index (col)=2 ("disabled index (col)")) -> (element=w285:string)
        n83 = Fract/Exp String To Number(string=w285) -> (number=w284:dbl)  [unwired: 3 in, 1 out]
        n84 = Build Array(1.0, w284) -> (w278:dbl[])
        n85 = Build Array(w283, w283) -> (w282:dbl[])
        n86 = Build Array(w280, w280) -> (w279:dbl[])
        n87 = Bundle(w282, w278) -> (w277:cluster{dbl[], dbl[]})  [unwired: 1 in]
        n88 = Bundle(w279, w278) -> (w276:cluster{dbl[], dbl[]})  [unwired: 1 in]
        n89 = Build Array(w277, w276) -> (w274:cluster{dbl[], dbl[]}[])
        n90 = Bundle("Row"=w275, w274) -> (w273:cluster{"Row":i32, cluster{dbl[], dbl[]}[]})  [unwired: 1 in]
        "cluster roi" <- w273
      }
      event "custom": Value Change {
        n91 = event-data() -> ()  [unwired: 1 in, 6 out]
        n92 = call "roi custom.vi"("Table"=w304, "Error In"=w311, "Cluster roi in"=w310, "List ROI In"=w313, "Spectrum In"=w303) -> ("Error Out"=w312:errorcluster, "Cluster roi out"=w309:T2, "List ROI Out"=w308:dbl[][])  [unwired: 4 in]
        n93 = call "roi_selection.vi"("List Parameter Fit In"=w307, "List ROI In"=w308, "List Peaks"=w304, "Spectrum In"=w303) -> ("List Parameter Fit Out"=w306:dbl[][], "List ROI Out"=w305:dbl[][])  [unwired: 6 in]
      }
      event "Reset": Value Change {
        w321 = FALSE
        n94 = event-data() -> ()  [unwired: 1 in, 6 out]
        n95 = call <vilib>:"Destroy Cursor.vi"("cursor ID"=w325, "error in (no error)"=w328) -> ("error out"=w330:errorcluster)  [unwired: 8 in]
        n96 = call-poly <vilib>:"Set Cursor.vi"("error in (no error)"=w330, "icon"=u16 1 ("Cursor Icon")) -> ("error out"=w327:errorcluster, "previous cursor ID"=w326:refnum<k1>)  [unwired: 8 in]
        n97 = Unbundle(w334) -> ("Locations"=w336:dbl[], "Amplitudes"=w335:dbl[])
        n98 = for {
          tunnel: w336 -> [w344] mode=indexing
          tunnel: w335 -> [w343] mode=indexing
          tunnel: T4 {"Name"="", "Color"=16776704, "Style"=4, "Point Style"=13, "Name Visible"=FALSE, "Allow Drag"=TRUE, "Cursor Mode"=0, "Plot"=0, "Index"=0, "Position"={"X"=0.0, "Y"=0.0}, "X Scale"=0, "Y Scale"=0, "Watch Plots"=[], "Watch All Plots"=FALSE, "Plot Area"=0, "Label Offset"={"X"=0.0, "Y"=0.0}} -> [w342]
          tunnel: [w338] -> w332 mode=indexing
          i -> [w345]
          (unwired) cluster{"X":dbl, "Y":dbl} {"X"=0.0, "Y"=0.0} ("XY")
          n99 = Bundle("Numeric Control"=w344, "Numeric"=w343) -> (w339:cluster{"Numeric Control":dbl, "Numeric":dbl})  [unwired: 1 in]
          n100 = Format Into String(format string="Cursor %d", w345) -> (resulting string=w341:string)  [unwired: 2 in, 1 out]
          n101 = Bundle By Name(cluster=w342, "Name"=w341, "Position"=w339, "Color"=u32 1985280) -> (w338:T4)
        }
        n102 = property on="Spectrum" class="XYGraph (strict)"("CrsrList"=w332) -> ()  [unwired: 2 in, 2 out]
        n103 = local write "removing"(FALSE ("removing")) -> ()
      }
      event "eval": Value Change {
        n104 = event-data() -> ()  [unwired: 1 in, 6 out]
        n105 = call "roi_selection.vi"("Starting Evaluate?"="eval", "List Parameter Fit In"=w348, "List ROI In"=w349, "List Peaks"=w360, "Spectrum In"=w361) -> ("List Parameter Fit Out"=w350:dbl[][], "List ROI Out"=w359:dbl[][])  [unwired: 5 in]
      }
      event "Save": Value Change {
        n106 = event-data() -> ()  [unwired: 1 in, 6 out]
        n107 = Format Into String(format string="%s_table_ROI.dat", w368) -> (resulting string=w378:string)  [unwired: 2 in, 1 out]
        n108 = Format Into String(format string="%s_table_peaks.dat", w368) -> (resulting string=w377:string)  [unwired: 2 in, 1 out]
        n109 = Build Path(base path=w362, name or relative path=w377) -> (appended path=w372:path)
        n110 = Build Path(base path=w362, name or relative path=w378) -> (appended path=w376:path)
        n111 = call-poly <vilib>:"Write Delimited Spreadsheet.vi"("file path (dialog if empty)"=w376, "2D data"=w375, "error in (no error)"=w374) -> ("error out"=w373:errorcluster)  [unwired: 11 in, 1 out]
        n112 = call-poly <vilib>:"Write Delimited Spreadsheet.vi"("file path (dialog if empty)"=w372, "2D data"=w371, "error in (no error)"=w373) -> ("error out"=w365:errorcluster)  [unwired: 11 in, 1 out]
        n113 = Format Into String(format string="%s_list_parameters_fit.dat", w368) -> (resulting string=w367:string)  [unwired: 2 in, 1 out]
        n114 = Build Path(base path=w362, name or relative path=w367) -> (appended path=w366:path)
        n115 = call-poly <vilib>:"Write Delimited Spreadsheet.vi"("file path (dialog if empty)"=w366, "2D data"=w363, "error in (no error)"=w365) -> ("error out"=w364:errorcluster)  [unwired: 11 in, 1 out]
      }
      event "Open": Value Change {
        n116 = event-data() -> ()  [unwired: 1 in, 6 out]
        n117 = property on="Spectrum" class="XYGraph (strict)"(error in=w398, "CrsrList"=T3 [] ("Cursor List")) -> (error out=w399:errorcluster)  [unwired: 1 in, 1 out]
        n118 = call-poly <vilib>:"Read Delimited Spreadsheet.vi"("error in (no error)"=w399) -> ("new file path (Not A Path if cancelled)"=w393:path, "all rows"=w403:string[][], "error out"=w404:errorcluster)  [unwired: 9 in, 3 out]
        n119 = Strip Path(path=w393) -> (stripped path=w407:path, name=w409:string)
        n120 = Match Pattern(string=w409, regular expression="_table_" ("format string")) -> (before substring=w410:string)  [unwired: 1 in, 3 out]
        n121 = for {
          tunnel: w403 -> [w432] mode=indexing
          tunnel: T4 {"Name"="", "Color"=16776704, "Style"=4, "Point Style"=13, "Name Visible"=FALSE, "Allow Drag"=TRUE, "Cursor Mode"=0, "Plot"=0, "Index"=0, "Position"={"X"=0.0, "Y"=0.0}, "X Scale"=0, "Y Scale"=0, "Watch Plots"=[], "Watch All Plots"=FALSE, "Plot Area"=0, "Label Offset"={"X"=0.0, "Y"=0.0}} -> [w421]
          tunnel: [w420] -> w401 mode=indexing
          i -> [w419]
          n122 = Index Array(array=w432, index #1=1 ("index"), index #2=2 ("index")) -> (element #1=w429:string, element #2=w428:string)
          n123 = Fract/Exp String To Number(string=w429) -> (number=w423:dbl)  [unwired: 3 in, 1 out]
          n124 = Fract/Exp String To Number(string=w428) -> (number=w422:dbl)  [unwired: 3 in, 1 out]
          n125 = Bundle(w423, w422) -> (w427:cluster{dbl, dbl})  [unwired: 1 in]
          n126 = Format Into String(format string="Cursor %d", w419) -> (resulting string=w426:string)  [unwired: 2 in, 1 out]
          n127 = Bundle By Name(cluster=w421, "Name"=w426, "Position"=w427, "Color"=u32 1985280) -> (w420:T4)
        }
        n128 = Strip Path(path=w393) -> (stripped path=w397:path, name=w395:string)
        n129 = Format Into String(format string="%s_table_ROI.dat", w410) -> (resulting string=w408:string)  [unwired: 2 in, 1 out]
        n130 = Build Path(base path=w407, name or relative path=w408) -> (appended path=w406:path)
        n131 = Match Pattern(string=w395, regular expression="_table_" ("format string")) -> (before substring=w391:string)  [unwired: 1 in, 3 out]
        n132 = call-poly <vilib>:"Read Delimited Spreadsheet.vi"("file path (dialog if empty)"=w406, "error in (no error)"=w404) -> ("all rows"=w405:dbl[][], "error out"=w389:errorcluster)  [unwired: 8 in, 4 out]
        n133 = Format Into String(format string="%s_list_parameters_fit.dat", w391) -> (resulting string=w396:string)  [unwired: 2 in, 1 out]
        n134 = Build Path(base path=w397, name or relative path=w396) -> (appended path=w390:path)
        n135 = call-poly <vilib>:"Read Delimited Spreadsheet.vi"("file path (dialog if empty)"=w390, "error in (no error)"=w389) -> ("all rows"=w387:dbl[][], "error out"=w388:errorcluster)  [unwired: 8 in, 4 out]
      }
      event "mapping": Value Change {
        n136 = event-data() -> ()  [unwired: 1 in, 6 out]
        n137 = case shown="1" "mapping" {
          selector: "mapping" -> [w446 w448]
          frame 0, Default {
            n138 = property on="Spectrum" class="XYGraph (strict)"("YScale.Mapping Mode"=w446, "YScale.ScaleFit"=u8 1 ("Y Scale.Scale Fit")) -> ()  [unwired: 2 in, 2 out]
          }
          frame 1 {
            n139 = property on="Spectrum" class="XYGraph (strict)"("YScale.Mapping Mode"=w448, "YScale.ScaleFit"=u8 1 ("Y Scale.Scale Fit")) -> ()  [unwired: 2 in, 2 out]
          }
        }
      }
    }
  }
  "Peaks Out" <- w16
  n140 = property on="List ROI out" class="Arr (strict)"("Value"=w7) -> ()  [unwired: 2 in, 2 out]
  n141 = property on="List Parameter Fit Out" class="Arr (strict)"("Value"=w6) -> ()  [unwired: 2 in, 2 out]
  n142 = call <vilib>:"Destroy Cursor.vi"("cursor ID"=w29, "error in (no error)"=w31) -> ("error out"=→"Error Out":errorcluster)  [unwired: 8 in]
  n143 = property on="Table" class="Tbl (strict)"("Value"=w5) -> ()  [unwired: 2 in, 2 out]
  "Spectrum" <- "Spectrum In"
